vi "简单工厂设计模式DEMO.vi"() -> ()   [LabVIEW 2013]
uses:
  Operation_class/Operation.lvclass
  Factory_class/Factory.lvclass
  <vilib>/addons/_AddQ/G#Object/G#Object.lvclass
panel:
  in  "停止":bool
  out "# of objects killed":i32
  out "Output":string
  out "result":dbl
  in  "y":dbl
  in  "x":dbl
  in  "Operation":enum16{"Add", "Mul"}(ring)
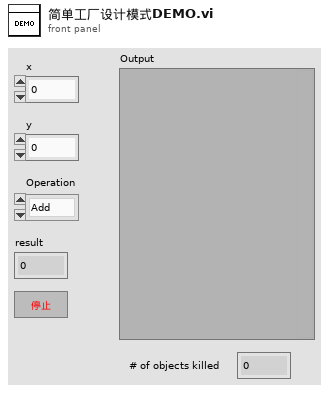
[diagram p1: front panel]
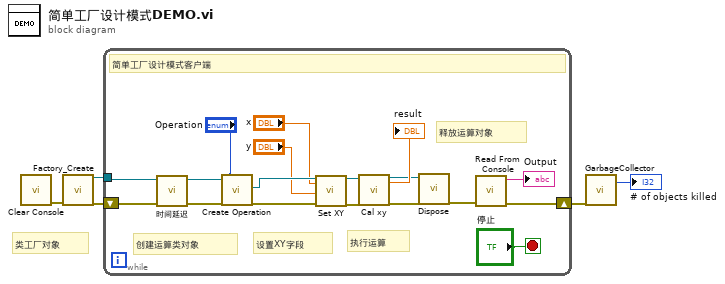
[diagram p0: block diagram]
diagram:
  # "类工厂对象"
  n1 = call "Clear Console.vi"() -> ("error out"=w3:errorcluster)  [unwired: 11 in]
  n2 = call "Factory_Create.vi"("error in (no error)"=w3) -> ("reference out"=w4:refnum<class "Factory.lvclass">, "error out"=w5:errorcluster)  [unwired: 17 in]
  n3 = while {
    shift-right: [w18] -> w2
    shift-left: w5 -> [w21]
    tunnel: w4 -> [w19]
    stop <- "停止" stop-if-true
    # "释放运算对象"
    # "执行运算"
    # "设置XY字段"
    # "创建运算类对象"
    # "简单工厂设计模式客户端"
    n4 = call "时间延迟"("error in (no error)"=w21) -> ("error out"=w20:errorcluster)  [unwired: 10 in]
    n5 = call "Create Operation.vi"("reference in"=w19, "error in (no error)"=w20, "Operation"="Operation") -> ("Operation"=w13:refnum<class "Operation.lvclass">, "error out"=w15:errorcluster)  [unwired: 14 in, 1 out]
    n6 = call "Set XY.vi"("reference in"=w13, "x"="x", "y"="y", "error in (no error)"=w15) -> ("reference out"=w10:refnum<class "Operation.lvclass">, "error out"=w14:errorcluster)  [unwired: 14 in]
    n7 = call-dynamic "Cal xy.vi"("reference in"=w10, "error in (no error)"=w14) -> ("reference out"=w7:refnum<class "Operation.lvclass">, "result"=→"result":dbl, "error out"=w8:errorcluster)  [unwired: 15 in]
    n8 = call-dynamic "Dispose.vi"("reference in"=w7, "error in (no error)"=w8) -> ("error out"=w6:errorcluster)  [unwired: 16 in, 1 out]
    n9 = call "Read From Console.vi"("error in (no error)"=w6) -> ("error out"=w18:errorcluster, "Output"=→"Output":string)  [unwired: 9 in]
  }
  n10 = call <vilib>:"GarbageCollector.vi"("error in (no error)"=w2) -> ("# of objects killed"=→"# of objects killed":i32)  [unwired: 16 in, 2 out]
